vi "CRYPreUpdate Sequence.vi"(0 "EventName":string="SequenceUpdate", 1 "Mode":string, 2 "StepName Arg3":string, 3 "Numeric":i32, 5 "Proper VI No":i32, 7 "AddSteps":refnum<vi>, 9 "Project View Step Name Identifier Arg1":string, 11 "Step flattened Arg2":string, 12 "AllChangeFlg":bool, 13 "Ref Variant":variant) -> ()   [LabVIEW 2013]
uses:
  CRYSystem/Typedef Control/CRYProjectViewCluster.ctl
  CRYProject/CRYProject Editor Global.vi
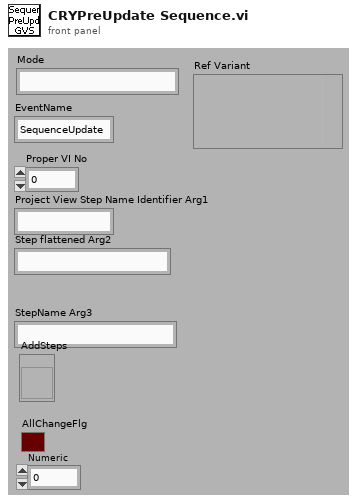
[diagram p1: front panel]
types:
  T1 = typedef "CRYProjectViewCluster.ctl" = cluster{"EventName":string, "Arg1":string, "Numeric":i32, "Proper VI No":i32, "AddSteps ":refnum<vi>, "Arg2":string, "Arg3":string, "Boolean":bool, "Mode":string, "Ref Variant":variant, "AllChangeFlg":bool}
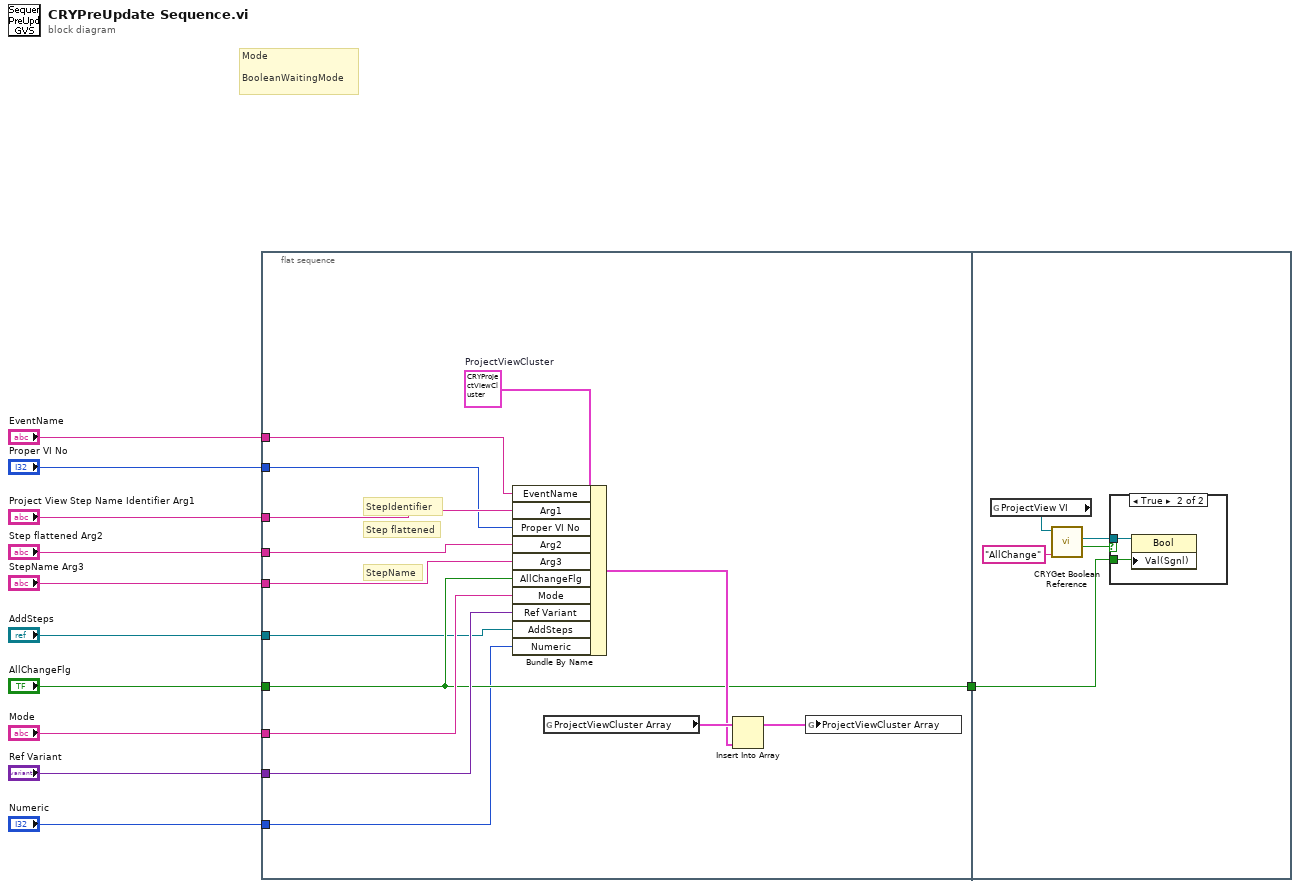
[diagram p0: block diagram]
diagram:
  # "Mode\n\nBooleanWaitingMode"
  n1 = flat-sequence {
    tunnel: "StepName Arg3" -> [w21]
    tunnel: "Project View Step Name Identifier Arg1" -> [w25]
    tunnel: "Step flattened Arg2" -> [w24]
    tunnel: "Proper VI No" -> [w23]
    tunnel: "EventName" -> [w22]
    tunnel: "Mode" -> [w16]
    tunnel: "Ref Variant" -> [w15]
    tunnel: "AllChangeFlg" -> [w14]
    tunnel: [w14] -> w1
    tunnel: "AddSteps" -> [w13]
    tunnel: "Numeric" -> [w12]
    tunnel: w1 -> [w26]
    frame #0 {
      w20 = T1 {"EventName"="", "Arg1"="", "Numeric"=0, "Proper VI No"=0, "AddSteps "=refnum, "Arg2"="", "Arg3"="", "Boolean"=FALSE, "Mode"="", "Ref Variant"=variant, "AllChangeFlg"=FALSE}  # ProjectViewCluster
      # "StepName"
      # "Step flattened"
      # "StepIdentifier"
      n2 = Bundle By Name(cluster=w20, "EventName"=w22, "Arg1"=w25, "Proper VI No"=w23, "Arg2"=w24, "Arg3"=w21, "AllChangeFlg"=w14, "Mode"=w16, "Ref Variant"=w15, "AddSteps"=w13, "Numeric"=w12) -> (w17:T1)
      n3 = global read "CRYProject Editor Global.vi" "ProjectViewCluster Array"() -> (w19:T1[])
      n4 = Insert Into Array(array=w19, new element=w17) -> (w18:T1[])  [unwired: 1 in]
      n5 = global write "CRYProject Editor Global.vi" "ProjectViewCluster Array"(w18) -> ()
    }
    frame #1 {
      n6 = global read "CRYProject Editor Global.vi" "ProjectView VI"() -> (w30:refnum<vi>)
      n7 = call "CRYGet Boolean Reference.vi"("Label Name"="AllChange", "VI Refnum"=w30) -> ("Exist?"=w28:bool, "Boolean Ref"=w27:refnum<vi>)  [unwired: 8 out]
      n8 = case shown="True" w28 {
        tunnel: w27 -> [_ w32]
        tunnel: w26 -> [_ w31]
        frame False {
        }
        frame True {
          n9 = property class="Bool"(reference=w32, "Val(Sgnl)"=w31) -> ()  [unwired: 1 in, 2 out]
        }
      }
    }
  }
